vi "Structure Handler.vi"() -> ()   [LabVIEW 2010] (continued)
.513237671579E-07   .564951247679E-07   .621875474984E-07   .684535380719E-07\n   .753508894551E-07   .829432179206E-07   .913005498212E-07   .100499967493E-06   .110626320242E-06\n   .121773006977E-06   .134042837705E-06   .147548981841E-06   .162416012071E-06   .178781053415E-06\n   .196795048071E-06   .216624147728E-06   .238451246178E-06   .262477666373E-06   .288925017504E-06\n   .318037239210E-06   .350082851806E-06   .385357433274E-06   .424186345884E-06   .466927737604E-06\n   .513975845980E-06   .565764635006E-06   .622771798513E-06   .685523167052E-06   .754597558918E-06\n   .830632120119E-06   .914328202545E-06   .100645783462E-05   .110787084417E-05   .121950269922E-05\n   .134238313919E-05   .147764567611E-05   .162653805357E-05   .179043376008E-05   .197084470305E-05\n   .216943516055E-05   .238803713959E-05   .262866728293E-05   .289354548047E-05   .318511535733E-05\n   .350606682774E-05   .385936092342E-05   .424825712563E-05   .467634345389E-05   .514756958921E-05\n   .566628333836E-05   .623727077631E-05   .686580043820E-05   .755767196958E-05   .831926968534E-05\n   .915762153277E-05   .100804640049E-04   .110963136049E-04   .122145455239E-04   .134454802607E-04\n   .148004789865E-04   .162920485386E-04   .179339570169E-04   .197413610551E-04   .217309459486E-04\n   .239210799391E-04   .263319840901E-04   .289859193303E-04   .319073924057E-04   .351233826543E-04\n   .386635917151E-04   .425607184965E-04   .468507619657E-04   .515733545831E-04   .567721294918E-04\n   .624951248914E-04   .687952293743E-04   .757306723900E-04   .833655644268E-04   .917704919735E-04\n   .101023172839E-03   .111209177984E-03   .122422726642E-03   .134767562225E-03   .148357917245E-03\n   .163319576369E-03   .179791047642E-03   .197924852956E-03   .217888949984E-03   .239868299087E-03\n   .264066590060E-03   .290708145179E-03   .320040016680E-03   .352334298733E-03   .387890676023E-03\n   .427039233419E-03   .470143553721E-03   .517604133365E-03   .569862149064E-03   .627403611879E-03\n   .690763949034E-03   .760533058090E-03   .837360882811E-03   .921963565285E-03   .101513023470E-02\n   .111773049960E-02   .123072271762E-02   .135516312450E-02   .149221591326E-02   .164316436368E-02\n   .180942313350E-02   .199255183450E-02   .219427002978E-02   .241647380359E-02   .266125407099E-02\n   .293091681294E-02   .322800544219E-02   .355532552753E-02   .391597212840E-02   .431336001852E-02\n   .475125710724E-02   .523382139980E-02   .576564187362E-02   .635178368709E-02   .699783818060E-02\n   .770997817641E-02   .849501913505E-02   .936048678149E-02   .103146918737E-01   .113668128506E-01\n   .125269871635E-01   .138064121687E-01   .152174565314E-01   .167737831718E-01   .184904848583E-01\n   .203842336354E-01   .224734453453E-01   .247784605712E-01   .273217433915E-01   .301280993745E-01\n   .332249142671E-01   .366424148226E-01   .404139531638E-01   .445763159812E-01   .491700596945E-01\n   .542398724605E-01   .598349635467E-01   .660094801087E-01   .728229507563E-01   .803407544570E-01\n   .886346122542E-01   .977830979381E-01   .107872162152E+00   .118995662400E+00   .131255889004E+00\n   .144764074182E+00   .159640868060E+00   .176016761568E+00   .194032431779E+00   .213838980399E+00\n   .235598030773E+00   .259481643242E+00   .285672002899E+00   .314360828291E+00   .345748444593E+00\n   .380042460821E+00   .417455988444E+00   .458205338955E+00   .502507141713E+00   .550574831420E+00\n   .602614468362E+00   .658819874780E+00   .719367098474E+00   .784408250325E+00   .854064805549E+00\n   .928420507861E+00   .100751406833E+01   .109133190169E+01   .117980118454E+01   .127278354258E+01\n   .137006966305E+01   .147137742340E+01   .157664611943E+01\n ae wavefunction\n   .535557091704E-08   .584615313749E-08   .637852560608E-08   .695650990210E-08   .758425806990E-08\n   .826628296378E-08   .900749126748E-08   .981321943576E-08   .106892728292E-07   .116419683371E-07\n   .126781808104E-07   .138053936581E-07   .150317539875E-07   .163661327113E-07   .178181900766E-07\n   .193984471166E-07   .211183635708E-07   .229904228708E-07   .250282248432E-07   .272465868411E-07\n   .296616540847E-07   .322910200607E-07   .351538579091E-07   .382710638186E-07   .416654135374E-07\n   .453617332187E-07   .493870859284E-07   .537709752675E-07   .585455677026E-07   .637459353389E-07\n   .694103210402E-07   .755804279757E-07   .823017358680E-07   .896238464348E-07   .976008607458E-07\n   .106291791475E-06   .115761013316E-06   .126078755115E-06   .137321637649E-06   .149573261301E-06\n   .162924848323E-06   .177475944810E-06   .193335187973E-06   .210621144868E-06   .229463229277E-06\n   .250002704098E-06   .272393777294E-06   .296804800206E-06   .323419577871E-06   .352438801904E-06\n   .384081617500E-06   .418587337205E-06   .456217315308E-06   .497256998019E-06   .542018166025E-06\n   .590841387595E-06   .644098702138E-06   .702196555972E-06   .765579014149E-06   .834731274431E-06\n   .910183511962E-06   .992515085916E-06   .108235914231E-05   .118040765045E-05   .128741691394E-05\n   .140421360120E-05   .153170134439E-05   .167086796061E-05   .182279335395E-05   .198865816282E-05\n   .216975322265E-05   .236748992100E-05   .258341152907E-05   .281920560166E-05   .307671754594E-05\n   .335796546920E-05   .366515642546E-05   .400070419254E-05   .436724872291E-05   .476767742530E-05\n   .520514844837E-05   .568311615361E-05   .620535898190E-05   .677600993702E-05   .739958992971E-05\n   .808104424844E-05   .882578244719E-05   .963972196691E-05   .105293358364E-04   .115017048293E-04\n   .125645744884E-04   .137264174648E-04   .149965016599E-04   .163849647036E-04   .179028953450E-04\n   .195624223894E-04   .213768118654E-04   .233605731714E-04   .255295750119E-04   .279011720082E-04\n   .304943429440E-04   .333298416879E-04   .364303619275E-04   .398207169443E-04   .435280357643E-04\n   .475819771328E-04   .520149628821E-04   .568624323930E-04   .621631199927E-04   .679593572815E-04\n   .742974025452E-04   .812277995842E-04   .888057684784E-04   .970916310060E-04   .106151273651E-03\n   .116056651362E-03   .126886335469E-03   .138726109423E-03   .151669616309E-03   .165819062365E-03\n   .181285981054E-03   .198192062573E-03   .216670054020E-03   .236864735810E-03   .258933980321E-03\n   .283049899139E-03   .309400085708E-03   .338188960618E-03   .369639227222E-03   .403993445736E-03\n   .441515734478E-03   .482493607363E-03   .527239957303E-03   .576095195662E-03   .629429558406E-03\n   .687645590114E-03   .751180817511E-03   .820510624648E-03   .896151342322E-03   .978663564752E-03\n   .106865570691E-02   .116678781619E-02   .127377565250E-02   .139039505069E-02   .151748657989E-02\n   .165596051352E-02   .180680212425E-02   .197107731740E-02   .214993861579E-02   .234463150841E-02\n   .255650117400E-02   .278699958957E-02   .303769303196E-02   .331026997863E-02   .360654941141E-02\n   .392848952388E-02   .427819682960E-02   .465793566447E-02   .507013807148E-02   .551741405100E-02\n   .600256215333E-02   .652858038310E-02   .709867737733E-02   .771628380971E-02   .838506396372E-02\n   .910892740586E-02   .989204067809E-02   .107388389144E-01   .116540372722E-01   .126426420512E-01\n   .137099613582E-01   .148616151513E-01   .161035444835E-01   .174420197380E-01   .188836476261E-01\n   .204353766962E-01   .221045010702E-01   .238986620996E-01   .258258475992E-01   .278943882806E-01\n   .301129509672E-01   .324905281293E-01   .350364232274E-01   .377602313017E-01   .406718142038E-01\n   .437812698306E-01   .470988947080E-01   .506351392801E-01   .544005552922E-01   .584057346980E-01\n   .626612395711E-01   .671775225433E-01   .719648373193E-01   .770331388378E-01   .823919726537E-01\n   .880503531153E-01   .940166299175E-01   .100298342637E+00   .106902062927E+00   .113833224167E+00\n   .121095938523E+00   .128692801551E+00   .136624684701E+00   .144890516314E+00   .153487051916E+00\n   .162408634982E+00   .171646949578E+00   .181190766703E+00   .191025686502E+00   .201133878922E+00\n   .211493825815E+00   .222080067897E+00   .232862960408E+00   .243808441743E+00   .254877819694E+00\n   .266027580335E+00   .277209224901E+00   .288369140290E+00   .299448509029E+00   .310383264646E+00\n   .321104098278E+00   .331536521915E+00   .341600992660E+00   .351213100691E+00   .360283821210E+00\n   .368719828095E+00   .376423865651E+00   .383295176394E+00   .389229988984E+00   .394122080847E+00\n   .397863441927E+00   .400345073211E+00   .401457947613E+00   .401094136245E+00   .399148068493E+00\n   .395517872662E+00   .390106751775E+00   .382824375227E+00   .373588286907E+00   .362325332199E+00\n   .348973096502E+00   .333481337937E+00   .315813392641E+00   .295947532026E+00   .273878254160E+00\n   .249617493172E+00   .223195730222E+00   .194662987245E+00   .164089681231E+00   .131567313019E+00\n   .972089612288E-01   .611495499793E-01   .235458591212E-01  -.154237513487E-01  -.555599253720E-01\n  -.966432190948E-01  -.138435344127E+00  -.180680758539E+00  -.223108628584E+00  -.265435190321E+00\n  -.307366500752E+00  -.348601411827E+00  -.388834295872E+00  -.427756778344E+00  -.465058000559E+00\n  -.500424206695E+00  -.533540096861E+00  -.564094053593E+00  -.591785950516E+00  -.616333933335E+00\n  -.637478529600E+00  -.654985045141E+00  -.668645509828E+00  -.678280660929E+00  -.683741885001E+00\n  -.684912828516E+00  -.681710402251E+00  -.674085030959E+00  -.662020139579E+00  -.645530959409E+00\n  -.624662775943E+00  -.599488740411E+00  -.570107351133E+00  -.536639690231E+00  -.499226481008E+00\n  -.458025014803E+00  -.413205983091E+00  -.364950242739E+00  -.313445539176E+00  -.258883212654E+00\n  -.201454915997E+00  -.141349372871E+00  -.787492042753E-01  -.138278434185E-01   .532534454775E-01\n   .122348422307E+00   .193328547557E+00   .266085373571E+00   .340532496791E+00   .416606938857E+00\n   .494269972861E+00   .573507668095E+00   .654331656637E+00   .736780660323E+00   .820923101590E+00\n   .906860813490E+00   .994733629756E+00   .108472460957E+01   .117706574281E+01   .127204411774E+01\n   .137000863656E+01   .147137742340E+01   .157664611943E+01\n End of Dataset\n"
  out "Bulk Options":T1(array[cluster])=[{"Structure Name"="CdTe Conv", "Lattice vector a"=[6.609392452716791, 0.0, 0.0], "Lattice vector b"=[0.0, 6.609392452716791, 0.0], "Lattice vector c"=[0.0, 0.0, 6.609392452716791], "Atoms Array"=[{"Atom Name"="Cd", "Positions (Direct)"=[[0.0, 0.0, 0.0], [0.0, 0.5, 0.5], [0.5, 0.0, 0.5], [0.5, 0.5, 0.0]], "Positions (Cartesian)"=[[0.0, 0.0, 0.0], [0.0, 3.3046962263583954, 3.3046962263583954], [3.3046962263583954, 0.0, 3.3046962263583954], [3.3046962263583954, 3.3046962263583954, 0.0]]}, {"Atom Name"="Te", "Positions (Direct)"=[[0.25, 0.25, 0.25], [0.75, 0.75, 0.25], [0.75, 0.25, 0.75], [0.25, 0.75, 0.75]], "Positions (Cartesian)"=[[1.6523481131791977, 1.6523481131791977, 1.6523481131791977], [4.957044339537593, 4.957044339537593, 1.6523481131791977], [4.957044339537593, 1.6523481131791977, 4.957044339537593], [1.6523481131791977, 4.957044339537593, 4.957044339537593]]}], "# of atoms"=8}, {"Structure Name"="111 Quasi-Bulk", "Lattice vector a"=[9.1641, 0.0, 0.0], "Lattice vector b"=[0.0, 7.93635, 0.0], "Lattice vector c"=[0.0, 0.0, 10.9], "Atoms Array"=[{"Atom Name"="Cd", "Positions (Direct)"=[[0.0386392660198839, 0.13013380691376078, 0.16738489560131178], [0.5386392660198832, 0.13013380691376078, 0.16738489560131178], [0.28863926601988393, 0.6301338069137602, 0.16738489560131178], [0.7886392660198832, 0.6301338069137602, 0.16738489560131178], [0.285711565948201, 0.2950238966446133, 0.5009960396727412], [0.7857115659482008, 0.2950238966446133, 0.5009960396727412], [0.0357115659482008, 0.7950238966446125, 0.5009960396727412], [0.5357115659482008, 0.7950238966446125, 0.5009960396727412], [0.0325958294469598, 0.46487896030108916, 0.8343605349746149], [0.5325958294469597, 0.46487896030108916, 0.8343605349746149], [0.2825958294469597, 0.9648789603010888, 0.8343605349746149], [0.7825958294469597, 0.9648789603010888, 0.8343605349746149]], "Positions (Cartesian)"=[[0.354094097732818, 1.0327874385000255, 1.8244953620542987], [4.936144097732812, 1.0327874385000255, 1.8244953620542987], [2.6451190977328185, 5.0009624385000215, 1.8244953620542987], [7.227169097732811, 5.0009624385000215, 1.8244953620542987], [2.6182893615059086, 2.341412902135477, 5.46085683243288], [7.200339361505907, 2.341412902135477, 5.46085683243288], [0.327264361505907, 6.309587902135471, 5.46085683243288], [4.909314361505906, 6.309587902135471, 5.46085683243288], [0.2987114406348843, 3.689442136585549, 9.094529831223303], [4.880761440634883, 3.689442136585549, 9.094529831223303], [2.5897364406348835, 7.6576171365855465, 9.094529831223303], [7.171786440634883, 7.6576171365855465, 9.094529831223303]]}, {"Atom Name"="Te", "Positions (Direct)"=[[0.2885476016109279, 0.29660400265422154, 0.24621241720575482], [0.7885476016109273, 0.29660400265422154, 0.24621241720575482], [0.03854760161092769, 0.7966040026542218, 0.24621241720575482], [0.5385476016109273, 0.7966040026542218, 0.24621241720575482], [0.035661094149161, 0.46186638195750324, 0.5797562346067128], [0.5356610941491612, 0.46186638195750324, 0.5797562346067128], [0.28566109414916063, 0.9618663819575034, 0.5797562346067128], [0.7856610941491612, 0.9618663819575034, 0.5797562346067128], [0.0325174374326621, 0.1313413350620399, 0.9129383313441972], [0.5325174374326627, 0.1313413350620399, 0.9129383313441972], [0.282517437432662, 0.6313413350620392, 0.9129383313441972], [0.7825174374326627, 0.6313413350620392, 0.9129383313441972]], "Positions (Cartesian)"=[[2.644279075922704, 2.3539531764648314, 2.683715347542728], [7.226329075922698, 2.3539531764648314, 2.683715347542728], [0.35325407592270247, 6.322128176464834, 2.683715347542728], [4.935304075922699, 6.322128176464834, 2.683715347542728], [0.3268018328923263, 3.665533260448431, 6.31934295721317], [4.908851832892328, 3.665533260448431, 6.31934295721317], [2.617826832892323, 7.633708260448433, 6.31934295721317], [7.199876832892327, 7.633708260448433, 6.31934295721317], [0.2979930483766587, 1.0423708045196205, 9.95102781165175], [4.880043048376663, 1.0423708045196205, 9.95102781165175], [2.5890180483766576, 5.010545804519615, 9.95102781165175], [7.171068048376664, 5.010545804519615, 9.95102781165175]]}], "# of atoms"=88}, {"Structure Name"="A Quasi-Bulk", "Lattice vector a"=[9.1641, 0.0, 0.0], "Lattice vector b"=[0.0, 7.93637, 0.0], "Lattice vector c"=[0.0, 0.0, 11.6], "Atoms Array"=[{"Atom Name"="Cd", "Positions (Direct)"=[[0.531704, 0.420048, 0.214582], [0.031704, 0.420048, 0.214582], [0.281704, 0.920046, 0.214582], [0.781703, 0.920046, 0.214582], [0.278968, 0.255395, 0.547757], [0.778967, 0.255395, 0.547757], [0.528968, 0.755394, 0.547757], [0.028968, 0.755394, 0.547757], [0.526702, 0.091167, 0.880998], [0.026702, 0.091167, 0.880998], [0.276702, 0.591165, 0.880998], [0.776701, 0.591165, 0.880998]], "Positions (Cartesian)"=[[4.872588626399999, 3.3336563457599997, 2.4891512], [0.2905386264, 3.3336563457599997, 2.4891512], [2.5815636264, 7.30182547302, 2.4891512], [7.1636044623, 7.30182547302, 2.4891512], [2.5564906487999997, 2.02690921615, 6.353981200000001], [7.1385314847, 2.02690921615, 6.353981200000001], [4.8475156488, 5.99508627978, 6.353981200000001], [0.2654656488, 5.99508627978, 6.353981200000001], [4.8267497982, 0.72353504379, 10.219576799999999], [0.24469979819999998, 0.72353504379, 10.219576799999999], [2.5357247982, 4.6917041710500005, 10.219576799999999], [7.1177656340999995, 4.6917041710500005, 10.219576799999999]]}, {"Atom Name"="Te", "Positions (Direct)"=[[0.531773, 0.086648, 0.127003], [0.031773, 0.086648, 0.127003], [0.281773, 0.586646, 0.127003], [0.781772, 0.586646, 0.127003], [0.529175, 0.421928, 0.460149], [0.029175, 0.421928, 0.460149], [0.279175, 0.921926, 0.460149], [0.779174, 0.921926, 0.460149], [0.276819, 0.257634, 0.793416], [0.776818, 0.257634, 0.793416], [0.526819, 0.757633, 0.793416], [0.026819, 0.757633, 0.793416]], "Positions (Cartesian)"=[[4.8732209493, 0.68767058776, 1.4732348], [0.2911709493, 0.68767058776, 1.4732348], [2.5821959493, 4.65583971502, 1.4732348], [7.1642367852, 4.65583971502, 1.4732348], [4.8494126175, 3.34857672136, 5.3377284], [0.26736261749999995, 3.34857672136, 5.3377284], [2.5583876174999998, 7.31674584862, 5.3377284], [7.1404284534, 7.31674584862, 5.3377284], [2.5367969979, 2.04467874858, 9.2036256], [7.1188378338, 2.04467874858, 9.2036256], [4.8278219979, 6.01285581221, 9.2036256], [0.24577199789999998, 6.01285581221, 9.2036256]]}], "# of atoms"=24}, {"Structure Name"="B Quasi-Bulk", "Lattice vector a"=[9.1641, 0.0, 0.0], "Lattice vector b"=[0.0, 7.93637, 0.0], "Lattice vector c"=[0.0, 0.0, 11.6], "Atoms Array"=[{"Atom Name"="Cd", "Positions (Direct)"=[[0.283771, 0.252605, 0.232263], [0.783771, 0.252605, 0.232263], [0.033771, 0.752605, 0.232263], [0.533771, 0.752605, 0.232263], [0.033055, 0.418321, 0.565266], [0.533055, 0.418321, 0.565266], [0.283055, 0.918321, 0.565266], [0.783055, 0.918321, 0.565266], [0.03471, 0.084002, 0.898841], [0.53471, 0.084002, 0.898841], [0.28471, 0.584002, 0.898841], [0.78471, 0.584002, 0.898841]], "Positions (Cartesian)"=[[2.6005058210999996, 2.0047667438500003, 2.6942508], [7.182555821099999, 2.0047667438500003, 2.6942508], [0.3094808211, 5.9729517438499995, 2.6942508], [4.8915308211, 5.9729517438499995, 2.6942508], [0.3029193255, 3.31995023477, 6.557085600000001], [4.884969325499999, 3.31995023477, 6.557085600000001], [2.5939443255, 7.28813523477, 6.557085600000001], [7.175994325499999, 7.28813523477, 6.557085600000001], [0.31808591099999994, 0.66667095274, 10.4265556], [4.900135911, 0.66667095274, 10.4265556], [2.609110911, 4.634855952740001, 10.4265556], [7.191160911, 4.634855952740001, 10.4265556]]}, {"Atom Name"="Te", "Positions (Direct)"=[[0.033593, 0.085908, 0.144634], [0.533593, 0.085908, 0.144634], [0.283593, 0.585908, 0.144634], [0.783593, 0.585908, 0.144634], [0.283028, 0.251763, 0.4777], [0.783028, 0.251763, 0.4777], [0.033028, 0.751763, 0.4777], [0.533028, 0.751763, 0.4777], [0.034563, 0.417433, 0.810969], [0.534563, 0.417433, 0.810969], [0.284563, 0.917433, 0.810969], [0.784563, 0.917433, 0.810969]], "Positions (Cartesian)"=[[0.30784961129999994, 0.68179767396, 1.6777544000000002], [4.8898996113, 0.68179767396, 1.6777544000000002], [2.5988746113, 4.64998267396, 1.6777544000000002], [7.180924611299999, 4.64998267396, 1.6777544000000002], [2.5936968948, 1.99808432031, 5.54132], [7.175746894799999, 1.99808432031, 5.54132], [0.3026718948, 5.9662693203099995, 5.54132], [4.884721894799999, 5.9662693203099995, 5.54132], [0.3167387883, 3.31290273821, 9.407240400000001], [4.8987887883, 3.31290273821, 9.407240400000001], [2.6077637882999998, 7.281087738210001, 9.407240400000001], [7.1898137882999995, 7.281087738210001, 9.407240400000001]]}], "# of atoms"=24}]
  in  "Input Structure File":path=path "C:/Users/Chris/Documents/Ab-initio/VASP Calc/Batch13_20130801/1_A13B_utwin/POSCAR"
  in  "Tab Control":enum32{"Draw Screen"}(tab)
  out "Scene Display":refnum<vi>(3d-picture)
  in  "Scale":dbl(slide)=0.03473491773308958 scale=0.0..0.2
  in  "Atom Size":dbl=0.75
  in  "Options":cluster{"Border?":bool, "Bonds?":bool}
  in  "Auto-Setup Camera":bool=TRUE
  in  "Load in VESTA":bool
  # "Get all results where"
  # "where"
  # "between these dates"
  # "Interface not complete"
  # "Supercell"
  # "Use Draw Box"
  # "Prickle Structure"
  # "Re-orient Crystal"
  # "Lock"
  # "Use Current Structure"
  # "Generates a README file which VASP Helper will interpret"
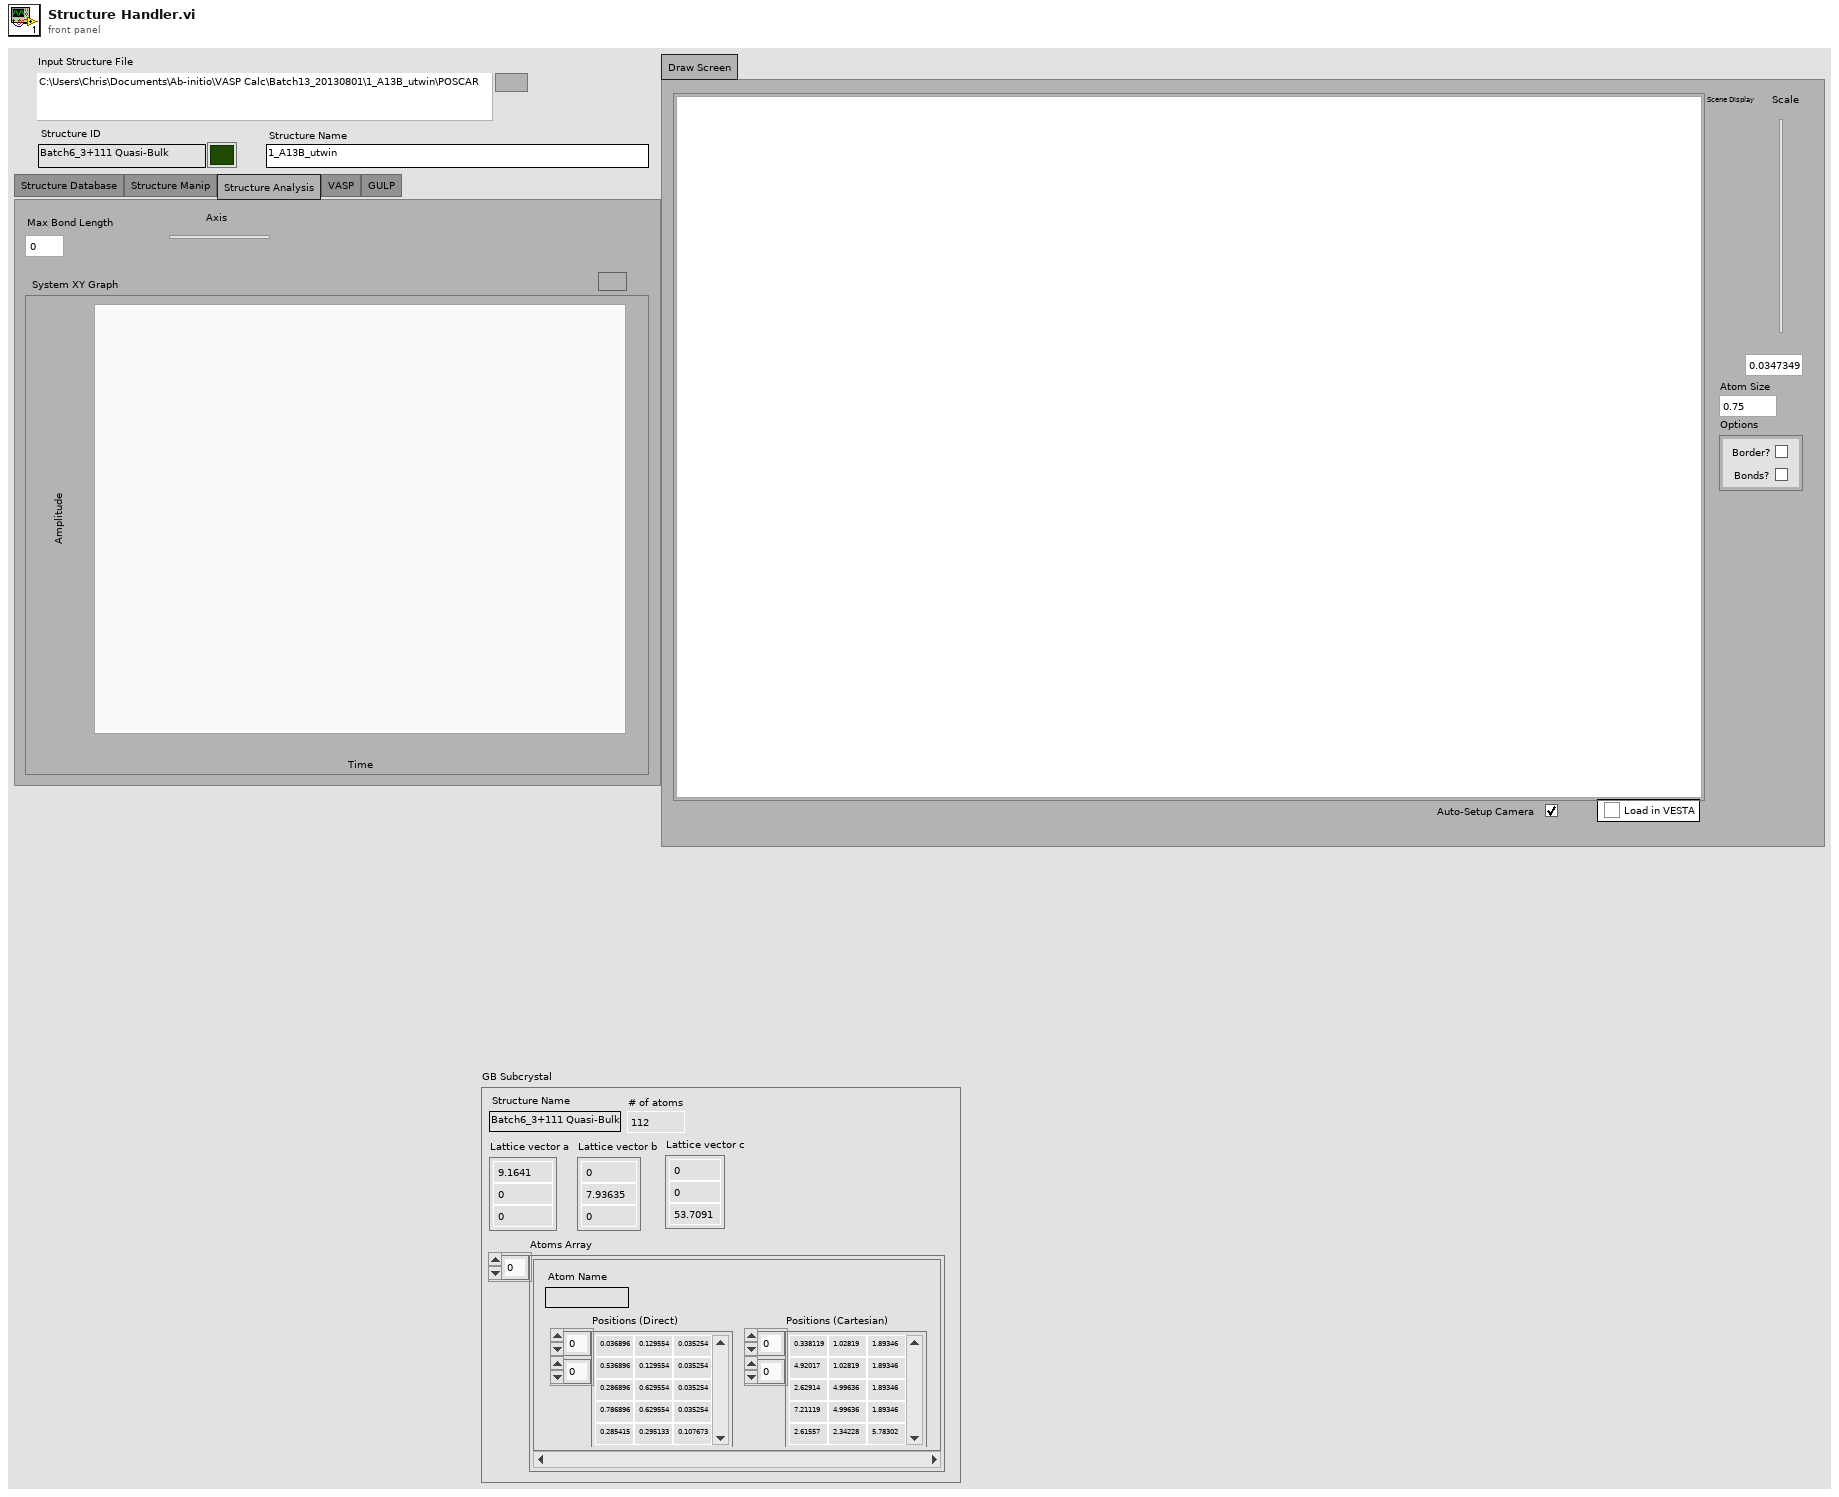
[diagram p1: front panel]
types:
  T1 = cluster{"Structure Name":string, "Lattice vector a":dbl[], "Lattice vector b":dbl[], "Lattice vector c":dbl[], "Atoms Array":cluster{"Atom Name":string, "Positions (Direct)":dbl[][], "Positions (Cartesian)":dbl[][]}[], "# of atoms":i32}[]
  T2 = typedef "LV3DPointTypeDef.ctl" = cluster{"X":sgl, "Y":sgl, "Z":sgl}
  T3 = cluster{"Structure Name":string, "Lattice vector a":dbl[], "Lattice vector b":dbl[], "Lattice vector c":dbl[], "Atoms Array":cluster{"Atom Name":string, "Positions (Direct)":dbl[][], "Positions (Cartesian)":dbl[][]}[], "# of atoms":i32}
  T4 = enum32{"Structure Database", "Structure Manip", "Structure Analysis", "VASP", "GULP"}
  T5 = cluster{"Sample Check box":bool, "Sample Comparison Type":string, "Sample Name":string, "Logical Sample-Lot ":string, "LotID Checkbox":bool, "Lot Comparison Type":string, "LotID Name":string, "Logical Lot-Date":string, "Date Checkbox":bool, "Start Date":timestamp, "End Date":timestamp, "1st search column name":string, "2nd search column name":string}
  T6 = cluster{"Defect Dimention":i8, "Defect Type":string, "Intrinsic or Extrinsic":string, "Comments":string}
  T7 = enum32{"Add, Crop Rotate", "Add 0D defects", "Create GB Manual", "Twins", "Structure"}
  T8 = enum32{"Pad with bulk", "Supercell", "Crop", "Remove Collisions", "Rotate", "Translate"}
  T9 = typedef "NI_Matrix.lvlib/RealMatrix.ctl" = dbl[][]
  T10 = enum32{"POSCAR", "POTCAR", "INCAR", "KPOINTS", "README", "JobScript"}
  T11 = enum32{"Gamma Centered Monkhurst-Pack", "Monkhurst-Pack"}
  T12 = cluster{"Start":dbl, "End":dbl, "Step or #pts":dbl, "Style":enum16{"Linear Step", "Linear Pts", "Log Pts"}, "Parameter":string}[]
  T13 = cluster{"Email at Beginning?":bool, "Email at End?":bool, "Email when aborted?":bool}
  T14 = cluster{"Number of Nodes":i32, "Processors per node":i32}
  T15 = cluster{"Lattice Vector Type":enum16{"Vectors", "Cell"}, "DoF to Allow Relaxation?":i32[]}
  T16 = cluster{"Potential Used":string, "Potential Details":cluster{"Atom 1":string, "Atom 2":string, "Parameters":dbl[], "Range Min (A)":dbl, "Range Max (A)":dbl}[]}
  T17 = typedef "NI_Database_API.lvlib/Conn ObjectReference.ctl" = refnum<k1>
  T18 = typedef "NI_Database_API.lvlib/Rec ObjectReference.ctl" = refnum<k1>
  T19 = cluster{"Lattice vector b[0]":dbl, "Lattice vector b[1]":dbl, "Lattice vector b[2]":dbl}
  T20 = cluster{"Atom Name":string, "Positions (Direct)":dbl[][], "Positions (Cartesian)":dbl[][]}[]
  T21 = cluster{"norm":dbl, "norm":dbl, "norm":dbl, "norm":dbl, "norm":dbl, "norm":dbl}
  T22 = cluster{"Rotation Axis[0]":dbl, "Rotation Axis[1]":dbl, "Rotation Axis[2]":dbl}
  T23 = cluster{"Atom Name":string, "Positions (Direct)":dbl[][], "Positions (Cartesian)":dbl[][]}
  T24 = typedef "LVPoint32TypeDef.ctl" = cluster{"Horizontal":i32, "Vertical":i32}
  T25 = cluster{"[0]":string, "[1]":string, "[2]":string, "[3]":string, "[4]":string, "[5]":string, "[6]":string, "[7]":string, "[8]":string, "[9]":string, "[10]":string, "[11]":string, "[12]":string, "[13]":string, "[14]":string, "[15]":string, "[16]":string, "[17]":string}
  T26 = cluster{"Structure ID":string, "Atom Name":string, "Numeric":dbl, "Numeric":dbl, "Numeric":dbl}
  T27 = cluster{"Shift":bool, "Ctrl":bool, "Alt":bool, "Cmd":bool, "Opt":bool}
  T28 = typedef "LVPositionTypeDef.ctl" = cluster{"Left":i32, "Top":i32}
  T29 = cluster{"Replacement Atom":string, dbl[][], dbl[][]}
  T30 = cluster{"Replacement Atom":string, "Positions (Direct)":dbl[][], "Positions (Cartesian)":dbl[][]}[]
  T31 = cluster{"Bond Name":string, "Bond Center Position":dbl[], "Bond Length (A)":dbl}[]
  T32 = cluster{"Structure ID":string, "Lattice vector a":dbl[], "Lattice vector b":dbl[], "Lattice vector c":dbl[], "Atoms Array":cluster{"Atom Name":string, "Positions (Direct)":dbl[][], "Positions (Cartesian)":dbl[][]}[], "# of atoms":i32}
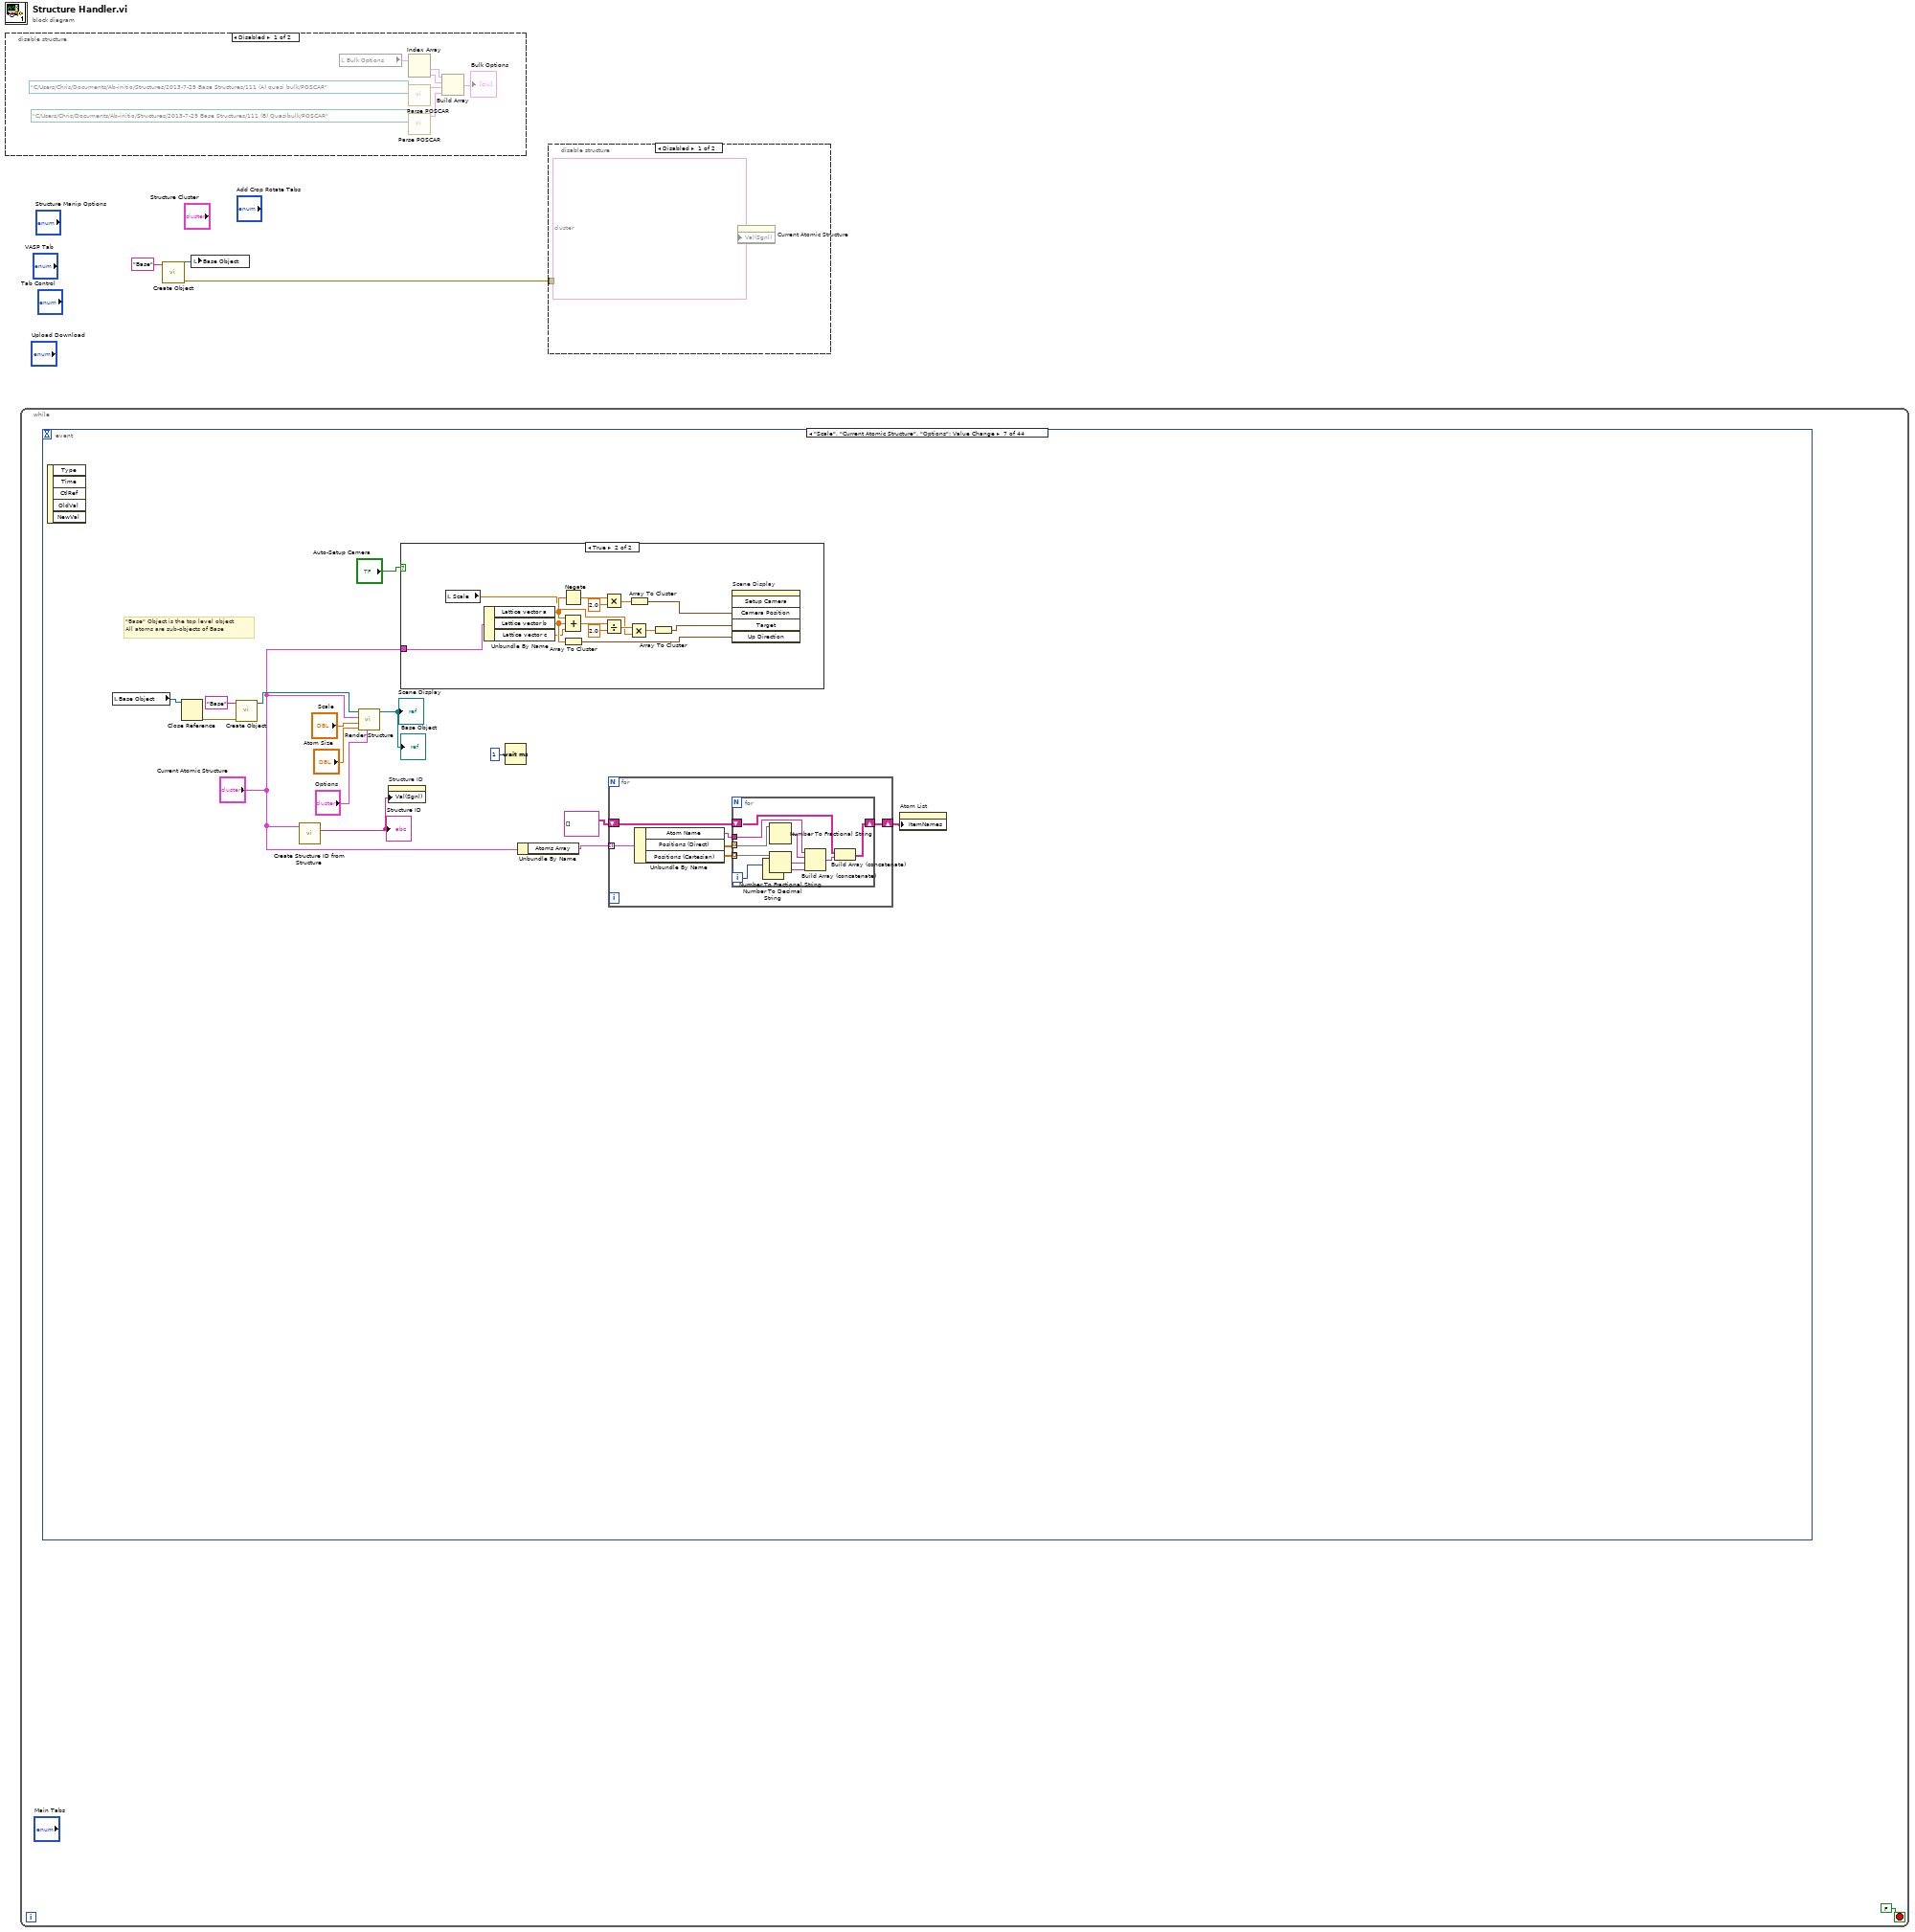
[diagram p0: block diagram]
diagram:
  n1 = disable-structure shown="Disabled" {
    frame Disabled {
      n2 = local read "Bulk Options"() -> (w11:T1)
      n3 = Index Array(array=w11) -> (element #1=w10:T3, element #2=w9:T3)  [unwired: 2 in]
      n4 = call "Parse POSCAR.vi"("POSCAR File"=path "C:/Users/Chris/Documents/Ab-initio/Structures/2013-7-29 Base Structures/111 (A) quasi bulk/POSCAR") -> ("Structure"=w7:T3)  [unwired: 7 in, 3 out]
      n5 = call "Parse POSCAR.vi"("POSCAR File"=path "C:/Users/Chris/Documents/Ab-initio/Structures/2013-7-29 Base Structures/111 (B) Quasibulk/POSCAR") -> ("Structure"=w6:T3)  [unwired: 7 in, 3 out]
      n6 = Build Array(w10, w9, w7, w6) -> (→"Bulk Options":T1)
    }
    frame Enabled {
    }
  }
  n7 = while {
    stop <- FALSE stop-if-true
    n8 = event shown="[6] \"Scale\", \"Current Atomic Structure\", \"Options\": Value Change" {
      selector: _ -> [_ _ _ _ _ _ _ _ _ _ _ _ _ _ _ _ _ _ _ _ _ _ _ _ _ _ _ _ _ _ _ _ _ _ _ _ _ _ _ _ _ _ _ _]
      dyn-events: _ -> [_ _ _ _ _ _ _ _ _ _ _ _ _ _ _ _ _ _ _ _ _ _ _ _ _ _ _ _ _ _ _ _ _ _ _ _ _ _ _ _ _ _ _ _]
      timeout: _ -> [_ _ _ _ _ _ _ _ _ _ _ _ _ _ _ _ _ _ _ _ _ _ _ _ _ _ _ _ _ _ _ _ _ _ _ _ _ _ _ _ _ _ _ _]
      event Timeout {
        n9 = event-data() -> ()  [unwired: 1 in, 2 out]
      }
      event "Main Tabs": Value Change {
        n10 = event-data() -> ("NewVal"=w13:T4)  [unwired: 1 in, 4 out]
        n11 = case shown="\"VASP\"" w13 {
          frame "Structure Database" {
            n12 = local read "Database UDL"() -> (w16:path)
